vi "AES Decrypt.vi"(5 "Key":u8[](array[numeric]), 7 "IV":u8[](array[numeric]), 8 "error in (no error)":errorcluster, 10 "encrypted_data":u8[](array[numeric]), 11 "AES in":refnum<class "AES.lvclass">) -> (0 "error out":errorcluster, 2 "data":string, 3 "AES out":refnum<class "AES.lvclass">)   [LabVIEW 2021, in "AES.lvclass"]
uses:
  AES.lvclass
  AES.lvclass/AES.ctl
  System.Core
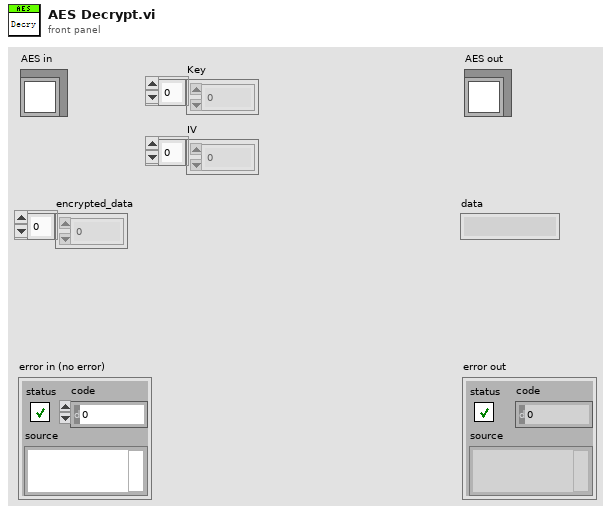
[diagram p1: front panel]
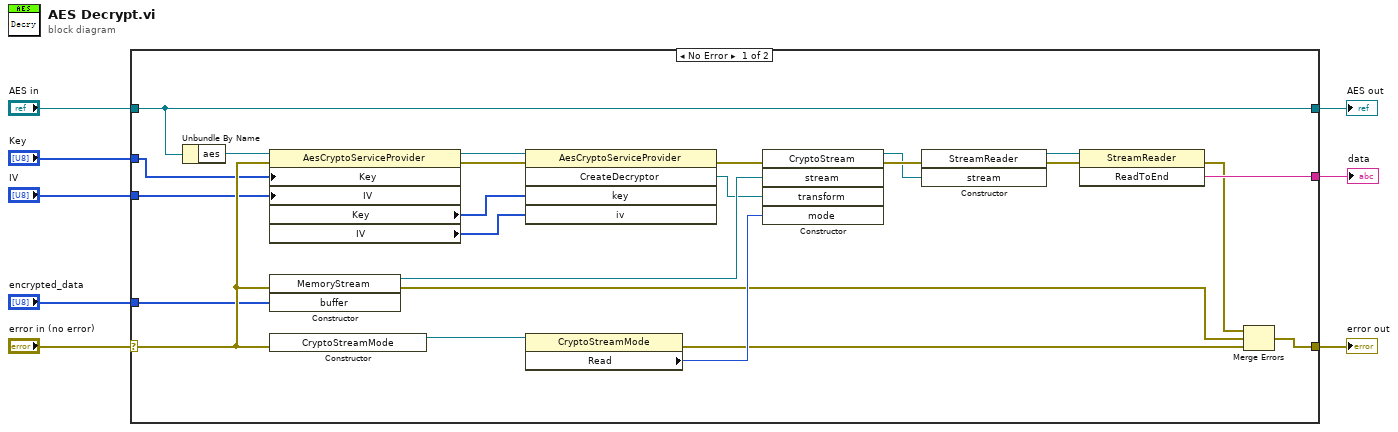
[diagram p0: block diagram]
diagram:
  n1 = case shown="No Error" "error in (no error)" {
    selector: "error in (no error)" -> [w16 w34]
    tunnel: [w9 w34] -> w7
    tunnel: [w32 w33] -> w5
    tunnel: "AES in" -> [w32 w33]
    tunnel: [w20 _] -> w4
    tunnel: "encrypted_data" -> [w15 _]
    tunnel: "Key" -> [w14 _]
    tunnel: "IV" -> [w13 _]
    frame No Error {
      n2 = Unbundle By Name(w32) -> ("aes"=w27:refnum<k24>)
      n3 = property class="AesCryptoServiceProvider"(reference=w27, error in=w16, "Key"=w14, "IV"=w13) -> (reference out=w30:refnum<k24>, error out=w31:errorcluster, "Key"=w29:u8[], "IV"=w28:u8[])
      n4 = constructor class="MemoryStream" ("AliceEntschlüsselt")(error in=w16, "buffer"=w15) -> (reference out=w19:refnum<k24>, error out=w11:errorcluster)  [unwired: 2 in, 2 out]
      n5 = constructor class="CryptoStreamMode" ("AliceEntschlüsselt")(error in=w16) -> (reference out=w26:refnum<k24>)  [unwired: 2 in, 2 out]
      n6 = invoke class="AesCryptoServiceProvider" method="CreateDecryptor"(reference=w30, error in=w31, "key"=w29, "iv"=w28) -> (error out=w25:errorcluster, "CreateDecryptor"=w17:refnum<k24>)  [unwired: 1 in, 3 out]
      n7 = property class="CryptoStreamMode"(reference=w26) -> (error out=w12:errorcluster, "Read"=w24:i32)  [unwired: 1 in, 1 out]
      n8 = constructor class="CryptoStream" ("AliceEntschlüsselt")(error in=w25, "stream"=w19, "transform"=w17, "mode"=w24) -> (reference out=w18:refnum<k24>, error out=w23:errorcluster)  [unwired: 2 in, 4 out]
      n9 = constructor class="StreamReader" ("AliceEntschlüsselt")(error in=w23, "stream"=w18) -> (reference out=w21:refnum<k24>, error out=w22:errorcluster)  [unwired: 2 in, 2 out]
      n10 = invoke class="StreamReader" method="ReadToEnd"(reference=w21, error in=w22) -> (error out=w10:errorcluster, "ReadToEnd"=w20:string)  [unwired: 1 in, 1 out]
      n11 = Merge Errors(w10, w11, w12) -> (w9:errorcluster)
    }
    frame Error {
    }
  }
  "error out" <- w7
  "AES out" <- w5
  "data" <- w4
